vi "Blur Colour Image.vi"(8 "Kernel Size (3,5,7)":i32=7 min=3 max=7 step=2, 10 "Image Dest":T1, 11 "Image Src":T1) -> (3 "Image Dest Out":T1)   [LabVIEW 2012]
uses:
  <vilib>/vision/Image Controls.llb/IMAQ Image.ctl
  <vilib>/vision/NI_Vision_Development_Module.lvlib
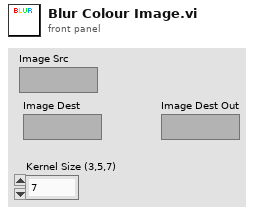
[diagram p1: front panel]
types:
  T1 = typedef "IMAQ Image.ctl" = refnum<image>
  T2 = typedef "Image Type" = u32
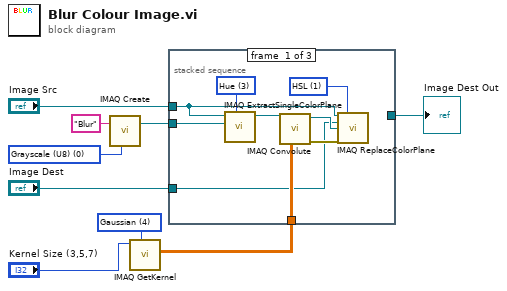
[diagram p0: block diagram]
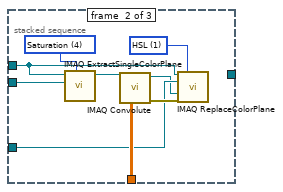
[diagram p2: hidden frame]
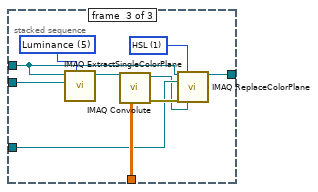
[diagram p3: hidden frame]
diagram:
  w4 = T2 0 items=["Grayscale (U8)", "Grayscale (I16)", "Grayscale (SGL)", "Complex (CSG)", "RGB (U32)", "HSL (U32)", "RGB (U64)", "Grayscale (U16)"] ("Image Type")
  w1 = u16 4 items=["Gradient"=1, "Laplacian"=2, "Smoothing"=3, "Gaussian"=4] ("Kernel Family")
  n1 = call "IMAQ Create"("Image Name"="Blur", "Image Type"=w4) -> ("New Image"=w5:T1)  [unwired: 3 in, 1 out]
  n2 = call "IMAQ GetKernel"("Kernel Family"=w1, "Kernel Size (3,5,...)"="Kernel Size (3,5,7)") -> ("Kernel"=w9:sgl[][])  [unwired: 6 in, 3 out]
  n3 = stacked-sequence {
    tunnel: "Image Src" -> [w11 w21 w31]
    tunnel: w5 -> [w17 w26 w36]
    tunnel: w9 -> [w15 w24 w34]
    tunnel: [_ _ w29] -> w8
    tunnel: "Image Dest" -> [w10 w20 w30]
    frame #0 {
      w12 = u16 1 items=["RGB", "HSL", "HSV", "HSI"] ("Color Mode")
      w18 = 3 items=["Red", "Green", "Blue", "Hue", "Saturation", "Luminance", "Value", "Intensity"] ("Color Plane")
      n4 = call "IMAQ ExtractSingleColorPlane"("Color Plane"=w18, "Image Dst"=w17, "Image Src"=w11) -> ("Image Dst Out"=w16:T1)  [unwired: 7 in, 1 out]
      n5 = call "IMAQ Convolute"("Kernel"=w15, "Image Src"=w16) -> ("error out"=w14:errorcluster, "Image Dst Out"=w13:T1)  [unwired: 8 in]
      n6 = call "IMAQ ReplaceColorPlane"("Image Src"=w11, "Color Mode"=w12, "Image Dst"=w10, "Red or Hue Plane"=w13, "error in (no error)"=w14) -> ()  [unwired: 9 in, 2 out]
    }
    frame #1 {
      w22 = u16 1 items=["RGB", "HSL", "HSV", "HSI"] ("Color Mode")
      w27 = 4 items=["Red", "Green", "Blue", "Hue", "Saturation", "Luminance", "Value", "Intensity"] ("Color Plane")
      n7 = call "IMAQ ExtractSingleColorPlane"("Color Plane"=w27, "Image Dst"=w26, "Image Src"=w21) -> ("Image Dst Out"=w25:T1)  [unwired: 7 in, 1 out]
      n8 = call "IMAQ Convolute"("Kernel"=w24, "Image Src"=w25) -> ("error out"=w23:errorcluster, "Image Dst Out"=w19:T1)  [unwired: 8 in]
      n9 = call "IMAQ ReplaceColorPlane"("Image Src"=w21, "Color Mode"=w22, "Image Dst"=w20, "Green or Sat Plane"=w19, "error in (no error)"=w23) -> ()  [unwired: 9 in, 2 out]
    }
    frame #2 {
      w32 = u16 1 items=["RGB", "HSL", "HSV", "HSI"] ("Color Mode")
      w37 = 5 items=["Red", "Green", "Blue", "Hue", "Saturation", "Luminance", "Value", "Intensity"] ("Color Plane")
      n10 = call "IMAQ ExtractSingleColorPlane"("Color Plane"=w37, "Image Dst"=w36, "Image Src"=w31) -> ("Image Dst Out"=w35:T1)  [unwired: 7 in, 1 out]
      n11 = call "IMAQ Convolute"("Kernel"=w34, "Image Src"=w35) -> ("error out"=w33:errorcluster, "Image Dst Out"=w28:T1)  [unwired: 8 in]
      n12 = call "IMAQ ReplaceColorPlane"("Image Src"=w31, "Color Mode"=w32, "Image Dst"=w30, "error in (no error)"=w33, "Blue or Luma or Val or Inten Plane"=w28) -> ("Image Dst Out"=w29:T1)  [unwired: 9 in, 1 out]
    }
  }
  "Image Dest Out" <- w8
